vi "Global FTT Display.vi"(8 "error in (no error)":errorcluster, 10 "W/R":bool, 11 "Display":T1={"Line.No"="", "Model"="", "Color"="", "UPH"=0.0, "Plan"=0.0, "Target Rate"=0.0, "Target "=0.0, "Actual"=0.0, "FTT"=0.0, "FTT Rate"=0.0, "Repaired"=0.0, "Reject"=0.0, "Ouline"=0.0, "Line State"="V254"}) -> (0 "error out":errorcluster, 3 "Display OUT":T1)   [LabVIEW 2014]
uses:
  Type'def/FTT Display Type.ctl
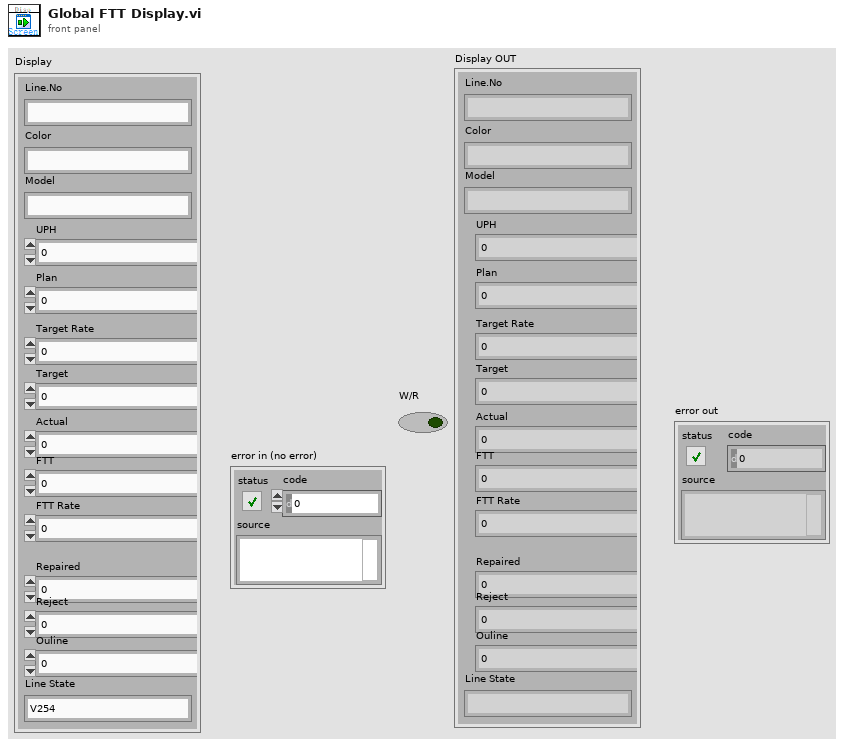
[diagram p1: front panel]
types:
  T1 = typedef "FTT Display Type.ctl" = cluster{"Line.No":string, "Model":string, "Color":string, "UPH":dbl, "Plan":dbl, "Target Rate":dbl, "Target ":dbl, "Actual":dbl, "FTT":dbl, "FTT Rate":dbl, "Repaired":dbl, "Reject":dbl, "Ouline":dbl, "Line State":string}
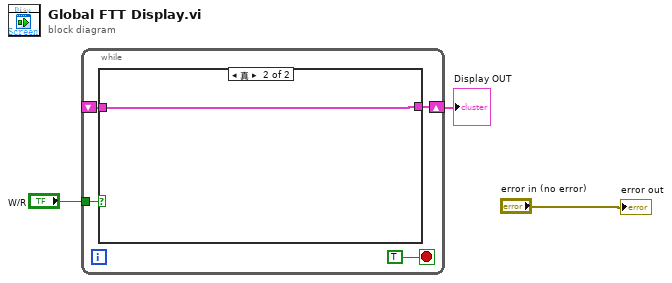
[diagram p0: block diagram]
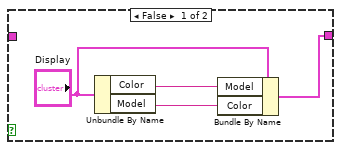
[diagram p2: hidden frame]
diagram:
  n1 = while {
    tunnel: "W/R" -> [w6]
    shift-right: [w5] -> w2
    shift-left: _ -> [w4]
    stop <- TRUE stop-if-true
    n2 = case shown="真" w6 {
      tunnel: [w10 w12] -> w5
      tunnel: w4 -> [_ w12]
      frame False {
        n3 = Unbundle By Name("Display") -> ("Color"=w9:string, "Model"=w8:string)
        n4 = Bundle By Name(cluster="Display", "Model"=w9, "Color"=w8) -> (w10:T1)
      }
      frame True {
      }
    }
  }
  "Display OUT" <- w2
  "error out" <- "error in (no error)"
